vi "modbusPort.vi"(10 "Modbus Port Settings":T1={"Tx Port"="ModbusPort1Tx", "Tx Data FIFO"="txModbusPort1FIFO", "Tx Internal FIFO"="txModbusPort1InternalFIFO", "Tx Telemetry FIFO"="txModbusPort1TelemetryFIFO", "Rx Port"="ModbusPort1Rx", "Rx Data FIFO"="rxModbusPort1FIFO", "Rx Telemetry FIFO"="txModbusPort1TelemetryFIFO", "Base Telemetry Address"=0, "Wait For Rx Frame Register"="WaitForPort1RxFrame", "IRQ Address"=0, "Trigger IRQ Register"="TriggerPort1IRQ", "Trigger IRQ Response Register"="TriggerPort1IRQ"}) -> ()   [LabVIEW 2015]
uses:
  DataTypes/ModbusPortSettings.ctl
  <vilib>/rvi/eio/common/nirviEmuTemplateMethod_errors.vi
  <vilib>/rvi/Emulation/niFpgaProcessEmulError.vi
  <vilib>/eio/EIONode/EIONode.xnode
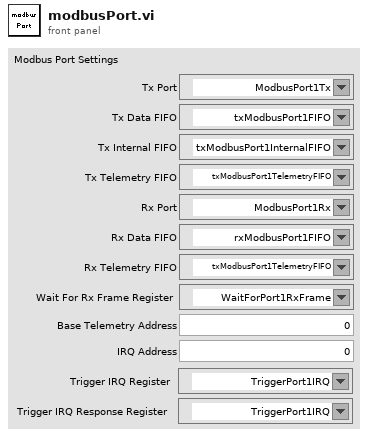
[diagram p1: front panel]
types:
  T1 = typedef "ModbusPortSettings.ctl" = cluster{"Tx Port":refnum<k21>, "Tx Data FIFO":refnum<k21>, "Tx Internal FIFO":refnum<k21>, "Tx Telemetry FIFO":refnum<k21>, "Rx Port":refnum<k21>, "Rx Data FIFO":refnum<k21>, "Rx Telemetry FIFO":refnum<k21>, "Base Telemetry Address":u32, "Wait For Rx Frame Register":refnum<k21>, "IRQ Address":u8, "Trigger IRQ Register":refnum<k21>, "Trigger IRQ Response Register":refnum<k21>}
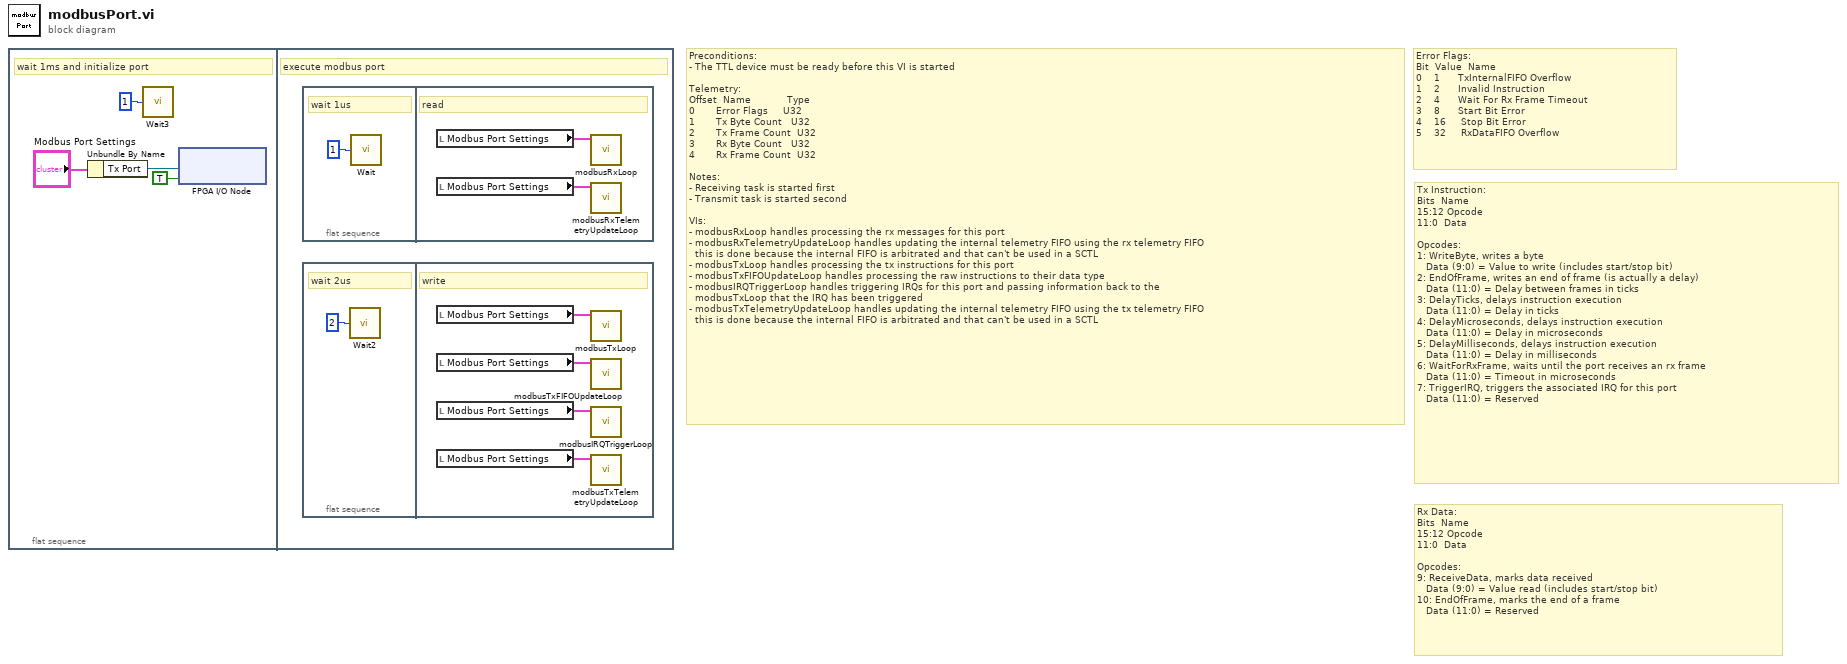
[diagram p0: block diagram]
diagram:
  # "Rx Data:\nBits  Name\n15:12 Opcode\n11:0  Data\n\nOpcodes:\n9: ReceiveData, marks data received\n   Data (9:0) = Value read (includes start/stop bit)\n10: EndOfFrame, marks the end of a frame\n   Data (11:0) = Reserved"
  # "Tx Instruction:\nBits  Name\n15:12 Opcode\n11:0  Data\n\nOpcodes:\n1: WriteByte, writes a byte\n   Data (9:0) = Value to write (includes start/stop bit)\n2: EndOfFrame, writes an end of frame (is actually a delay)\n   Data (11:0) = Delay between frames in ticks\n3: DelayTicks, delays instruction execution\n   Data (11:0) = Delay in ticks\n4: DelayMicroseconds, delays instruction execution\n   Data (11:0) = Delay in microseconds\n5: DelayMilliseconds, delays instruction execution\n   Data (11:0) = Delay in milliseconds\n6: WaitForRxFrame, waits until the port receives an rx frame\n   Data (11:0) = Timeout in microseconds\n7: TriggerIRQ, triggers the associated IRQ for this port\n   Data (11:0) = Reserved"
  # "Error Flags:\nBit  Value  Name\n0    1      TxInternalFIFO Overflow\n1    2      Invalid Instruction \n2    4      Wait For Rx Frame Timeout\n3    8      Start Bit Error\n4    16     Stop Bit Error\n5    32     RxDataFIFO Overflow"
  # "Preconditions:\n- The TTL device must be ready before this VI is started\n\nTelemetry:\nOffset  Name            Type\n0       Error Flags     U32         \n1       Tx Byte Count   U32\n2       Tx Frame Count  U32\n3       Rx Byte Count   U32\n4       Rx Frame Count  U32\n\nNotes:\n- Receiving task is started first\n- Transmit task is started second\n\nVIs:\n- modbusRxLoop handles processing the rx messages for this port\n- modbusRxTelemetryUpdateLoop handles updating the internal telemetry FIFO using the rx telemetry FIFO\n  this is done because the internal FIFO is arbitrated and that can't be used in a SCTL\n- modbusTxLoop handles processing the tx instructions for this port\n- modbusTxFIFOUpdateLoop handles processing the raw instructions to their data type\n- modbusIRQTriggerLoop handles triggering IRQs for this port and passing information back to the\n  modbusTxLoop that the IRQ has been triggered\n- modbusTxTelemetryUpdateLoop handles updating the internal telemetry FIFO using the tx telemetry FIFO\n  this is done because the internal FIFO is arbitrated and that can't be used in a SCTL"
  n1 = flat-sequence {
    frame #0 {
      # "wait 1ms and initialize port"
      n2 = Unbundle By Name("Modbus Port Settings") -> ("Tx Port"=w2:refnum<k21>)
      n3 = call "Wait3"("Count(mSec)"=u32 1 ("Count(Ticks)")) -> ()  [unwired: 1 out]
      n4 = xnode "FPGA I/O Node"("I/O Item"=TRUE, "FPGA I/O In"=w2) -> ()  [unwired: 1 out]
    }
    frame #1 {
      # "execute modbus port"
      n5 = flat-sequence {
        frame #0 {
          # "wait 1us"
          n6 = call "Wait"("Count(uSec)"=u32 1 ("Count(Ticks)")) -> ()  [unwired: 1 out]
        }
        frame #1 {
          # "read"
          n7 = local read "Modbus Port Settings"() -> (w12:T1)
          n8 = local read "Modbus Port Settings"() -> (w11:T1)
          n9 = call "modbusRxLoop.vi"("Modbus Port Settings"=w12) -> ()  [unwired: 11 in]
          n10 = call "modbusRxTelemetryUpdateLoop.vi"("Modbus Port Settings"=w11) -> ()  [unwired: 11 in]
        }
      }
      n11 = flat-sequence {
        frame #0 {
          # "wait 2us"
          n12 = call "Wait2"("Count(uSec)"=u32 2 ("Count(Ticks)")) -> ()  [unwired: 1 out]
        }
        frame #1 {
          # "write"
          n13 = local read "Modbus Port Settings"() -> (w9:T1)
          n14 = local read "Modbus Port Settings"() -> (w8:T1)
          n15 = local read "Modbus Port Settings"() -> (w7:T1)
          n16 = local read "Modbus Port Settings"() -> (w6:T1)
          n17 = call "modbusTxLoop.vi"("Modbus Port Settings"=w9) -> ()  [unwired: 11 in]
          n18 = call "modbusTxFIFOUpdateLoop.vi"("Modbus Port Settings"=w8) -> ()  [unwired: 11 in]
          n19 = call "modbusIRQTriggerLoop.vi"("Modbus Port Settings"=w7) -> ()  [unwired: 11 in]
          n20 = call "modbusTxTelemetryUpdateLoop.vi"("Modbus Port Settings"=w6) -> ()  [unwired: 11 in]
        }
      }
    }
  }
